vi "Create Power Data Plots.vi"(8 "error in (no error)":errorcluster) -> (0 "error out":errorcluster, 1 "DUT3 PowerData":T1, 2 "DUT2 PowerData":T1, 3 "DUT1 PowerData":T1, 4 "DUT4 PowerData":T1)   [LabVIEW 2019, in "Main.lvclass"]
doc: "Developed by Kevin Thompson\nkevin@thompsonengineering.net\n\nCopyright 2020\nThompson Engineering, LLC"
uses:
  Main.lvclass
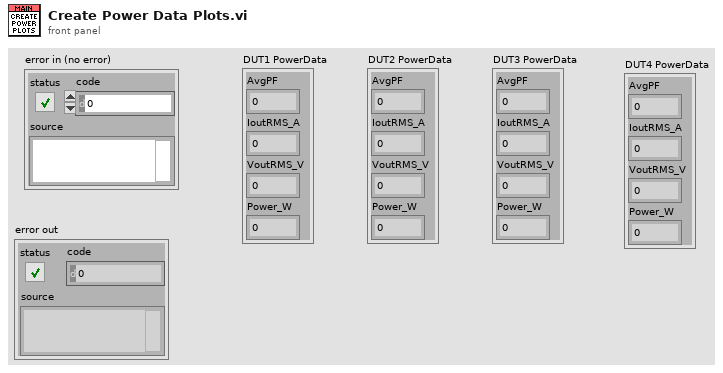
[diagram p1: front panel]
types:
  T1 = cluster{"AvgPF":dbl, "IoutRMS_A":dbl, "VoutRMS_V":dbl, "Power_W":dbl}
  T2 = typedef "TD MeasData--cluster.ctl" = cluster{"Timestamp":timestamp, "ESR_Ohm":dbl[], "DUT data":T3[], "DUT INVERTER data":cluster{"Raw ESR sum":dbl, "scaled raw ESR sum":dbl, "scaled and averaged raw ESR sum":dbl, "Total power":dbl}[]}
  T3 = typedef "InverterPhaseData--cluster.ctl" = cluster{"RawESR_Ohm":dbl, "TcompAvgESR_Ohm":dbl, "VoutRMS_V":dbl, "IoutRMS_A":dbl, "PF":dbl, "AvgPF":dbl, "Power_W":dbl, "AvgPower_W":dbl, "efficiency":dbl}
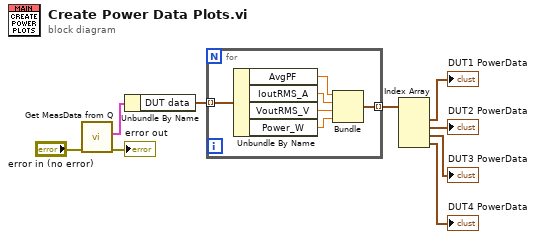
[diagram p0: block diagram]
diagram:
  n1 = call "Get MeasData from Q.vi"("error in (no error)"="error in (no error)") -> ("error out"=→"error out":errorcluster, "MeasData out"=w1:T2)  [unwired: 8 in, 1 out]
  n2 = Unbundle By Name(w1) -> ("DUT data"=w7:T3[])
  n3 = for {
    tunnel: w7 -> [w15] mode=indexing
    tunnel: [w10] -> w6 mode=indexing
    n4 = Unbundle By Name(w15) -> ("AvgPF"=w14:dbl, "IoutRMS_A"=w13:dbl, "VoutRMS_V"=w12:dbl, "Power_W"=w11:dbl)
    n5 = Bundle("AvgPF"=w14, "IoutRMS_A"=w13, "VoutRMS_V"=w12, "Power_W"=w11) -> (w10:T1)  [unwired: 1 in]
  }
  n6 = Index Array(array=w6) -> (element #1=→"DUT1 PowerData":T1, element #2=→"DUT2 PowerData":T1, element #3=→"DUT3 PowerData":T1, element #4=→"DUT4 PowerData":T1)  [unwired: 4 in]
